vi "BIO_f_ssl.vi"(8 "error in (no error)":errorcluster, 11 "SSL-Lib in":refnum<class "SSL-Lib.lvclass">) -> (0 "error out":errorcluster, 2 "*BIO_Method":u64, 3 "SSL-Lib out":refnum<class "SSL-Lib.lvclass">)   [LabVIEW 2013, in "OpenSSL Socket.lvlib" / "SSL-Lib.lvclass"]
uses:
  SSL-Lib.lvclass
  SSL-Lib.lvclass/SSL-Lib.ctl
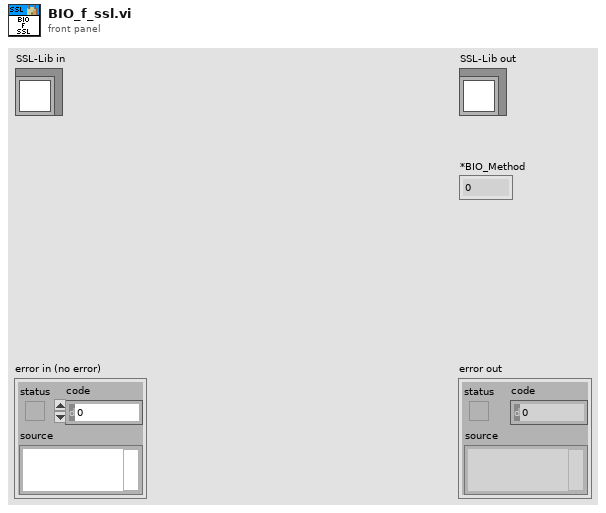
[diagram p1: front panel]
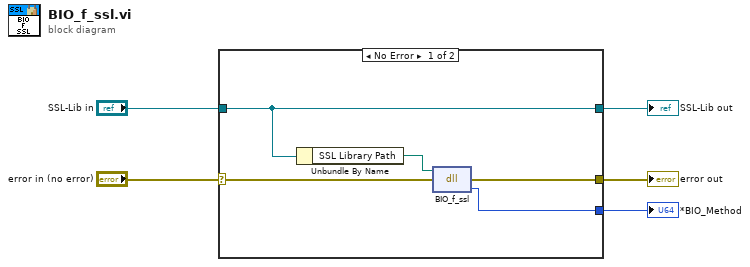
[diagram p0: block diagram]
diagram:
  n1 = case shown="No Error" "error in (no error)" {
    selector: "error in (no error)" -> [w10 w12]
    tunnel: [w7 w12] -> w4
    tunnel: [w9 w11] -> w2
    tunnel: "SSL-Lib in" -> [w9 w11]
    tunnel: [w6 _] -> w1
    frame No Error {
      n2 = Unbundle By Name(w9) -> ("SSL Library Path"=w8:path)
      n3 = dll-call lib="C:/Program Files (x86)/National Instruments/Shared/nissl/NIssleay32.dll" fn="BIO_f_ssl"(path in=w8, error in=w10) -> (error out=w7:errorcluster, "return type"=w6:u64)  [unwired: 1 in, 1 out]
    }
    frame Error {
    }
  }
  "error out" <- w4
  "SSL-Lib out" <- w2
  "*BIO_Method" <- w1
